vi "Get Request Type.vi"(8 "error in (no error)":errorcluster, 11 "SetInputVolume in":refnum<class "SetInputVolume.lvclass">) -> (0 "error out":errorcluster, 2 "Request Type":string, 3 "SetInputVolume out":refnum<class "SetInputVolume.lvclass">)   [LabVIEW 2022 SP3, in "obs-websocket-lv.lvlib" / "SetInputVolume.lvclass"]
uses:
  SetInputVolume.lvclass
  SetInputVolume.lvclass/SetInputVolume.ctl
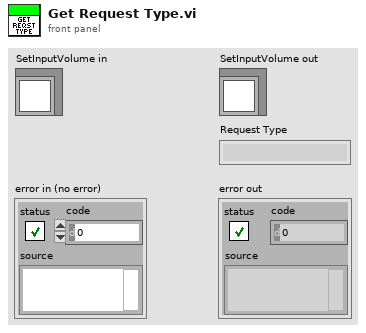
[diagram p1: front panel]
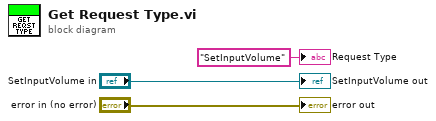
[diagram p0: block diagram]
diagram:
  "error out" <- "error in (no error)"
  "SetInputVolume out" <- "SetInputVolume in"
  "Request Type" <- "SetInputVolume" ("Request Type")
